vi "Current_SiPM_position.vi"(11 "Iteration":i32) -> (1 "SiPM_X":i32, 2 "Boolean 2":bool, 3 "Boolean":bool, 4 "SiPM_Y":i32)   [LabVIEW 2019]
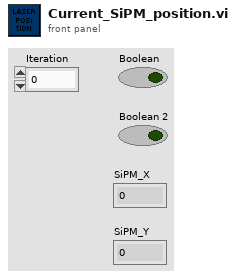
[diagram p1: front panel]
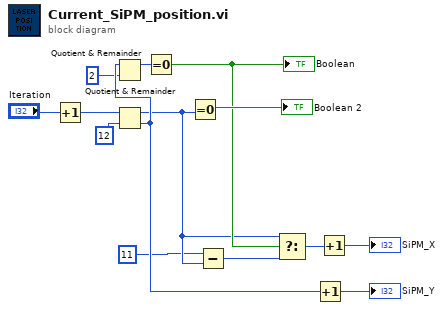
[diagram p0: block diagram]
diagram:
  n1 = Increment(x="Iteration") -> (x+1=w1:i32)
  n2 = Quotient & Remainder(x=w1, y=12) -> (x-y*floor(x/y)=w7:i32, floor(x/y)=w14:i32)
  n3 = Quotient & Remainder(x=w14, y=2) -> (x-y*floor(x/y)=w13:i32)  [unwired: 1 out]
  n4 = Equal To 0?(x=w13) -> (x = 0?=w8:bool)
  "Boolean" <- w8
  n5 = Equal To 0?(x=w7) -> (x = 0?=→"Boolean 2":bool)
  n6 = Subtract(x=11, y=w7) -> (x-y=w5:i32)
  n7 = Select(t=w7, s=w8, f=w5) -> (s? t:f=w4:i32)
  n8 = Increment(x=w14) -> (x+1=→"SiPM_Y":i32)
  n9 = Increment(x=w4) -> (x+1=→"SiPM_X":i32)
